vi "energy integration panel.vi"() -> ()   [LabVIEW 2017]
uses:
  control panel globals.vi
panel:
  out "fraction of energy lost/\nhalf cycle":dbl format="%_3e"
  out "adjusted energy/pulse":dbl format="%.3p"
  out "adjusted electromagnet energy":dbl format="%.3p"
  in  "coil adjustment":dbl=1.0
  out "starting energy":dbl format="%.3p"
  out "final energy":dbl format="%.3p"
  out "average energy":dbl format="%.3p"
  out "loss + change":dbl format="%.3p"
  out "energy change":dbl format="%.3p"
  out "electromagnet\nenergy":dbl format="%.3p"
  out "energy loss":dbl format="%.3p"
  out "elapsed time":dbl
  out "half cycles counted":dbl
  out "z0 from B0":dbl
  out "loss+change /hc":dbl format="%_3p"
  out "energy change/hc":dbl format="%_3p"
  out "electromagnet \nenergy/pulse":dbl format="%_3p"
  out "energy loss/hc":dbl format="%_3p"
  out "measurement":T1 {"Uavg" format="%_3p"; "Uloss" format="%_3p"; "Uloss_avg" format="%_3p"; "Upulse" format="%_3p"; "Upulse_avg" format="%_3p"; "DeltaU" format="%_3p"; "DeltaU_avg" format="%_3g"}
  in  "stop counting":bool
  in  "start counting":bool
  in  "lifetime with no drive (s)":dbl=1000.0
  in  "take snapshot":bool
  out "pulse statistics":T2 {"timing error" format="%#.3p"}
  # "totals"
  # "per 1/2 cycle"
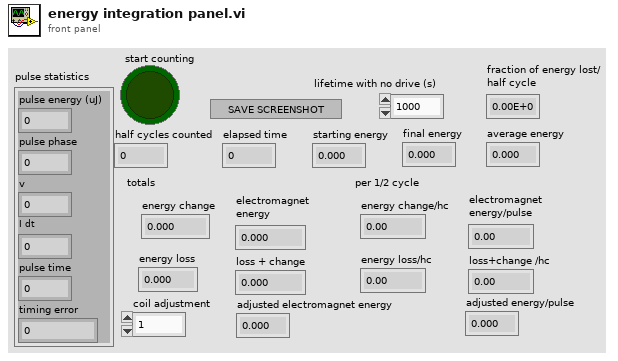
[diagram p1: front panel]
types:
  T1 = cluster{"Uavg":dbl, "Uloss":dbl, "Uloss_avg":dbl, "Upulse":dbl, "Upulse_avg":dbl, "DeltaU":dbl, "DeltaU_avg":dbl}
  T2 = cluster{"pulse energy (uJ)":sgl, "pulse phase":dbl, "v":dbl, "I dt":dbl, "pulse time":dbl, "timing error":dbl}
  T3 = cluster{"integrated pulse energy":dbl, "integrated amplitude squared":dbl, "integrated time":dbl, "integrated number of crossings":dbl, "starting amplitude squared":dbl, "final amplitude squared":dbl}
  T4 = cluster{"recent crossing":dbl, "prev crossing":dbl, "crossing-2":dbl, "number of crossings":i32, "period":dbl, "new crossing":bool, "new odd crossing":bool}
  T5 = typedef "magnetic field fit.ctl" = cluster{"a":dbl, "b":dbl, "theta":dbl, "scaling":dbl, "tilt_x":dbl, "tilt_y":dbl, "bx_offset":dbl, "by_offset":dbl, "bz_offset":dbl, "x_offset":dbl, "y_offset":dbl}
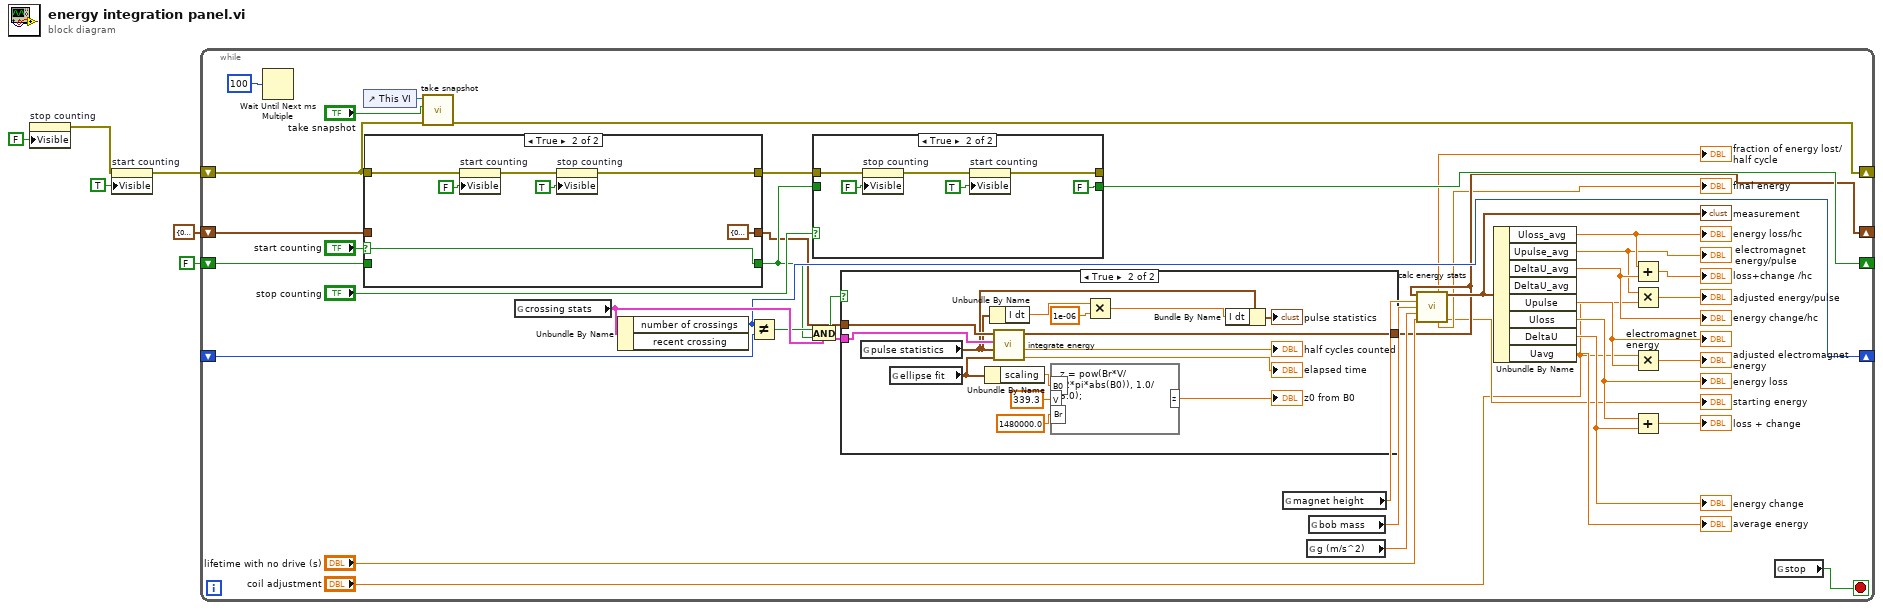
[diagram p0: block diagram]
diagram:
  n1 = property on="stop counting" class="Bool"("Visible"=FALSE) -> (error out=w4:errorcluster)  [unwired: 2 in, 1 out]
  n2 = property on="start counting" class="Bool"(error in=w4, "Visible"=TRUE) -> (error out=w3:errorcluster)  [unwired: 1 in, 1 out]
  n3 = while {
    shift-right: [w42] -> _
    shift-left: w3 -> [w36]
    shift-right: [w39] -> _
    shift-left: _ -> [w38]
    shift-right: [w15] -> _
    shift-left: T3 {"integrated pulse energy"=0.0, "integrated amplitude squared"=0.0, "integrated time"=0.0, "integrated number of crossings"=0.0, "starting amplitude squared"=0.0, "final amplitude squared"=0.0} ("integration cluster") -> [w33]
    shift-right: [w32] -> _
    shift-left: FALSE -> [w31]
    stop <- w45 stop-if-true
    n4 = Wait Until Next ms Multiple(millisecond multiple=u32 100) -> ()  [unwired: 1 out]
    n5 = control-ref of="This VI"() -> (w43:refnum<vi>)
    n6 = case shown="True" "start counting" {
      selector: "start counting" -> [_ w59]
      tunnel: [w57 T3 {"integrated pulse energy"=0.0, "integrated amplitude squared"=0.0, "integrated time"=0.0, "integrated number of crossings"=0.0, "starting amplitude squared"=0.0, "final amplitude squared"=0.0} ("integration cluster")] -> w28
      tunnel: w33 -> [w57 _]
      tunnel: w36 -> [w55 w62]
      tunnel: [w55 w60] -> w35
      tunnel: [w56 w59] -> w29
      tunnel: w31 -> [w56 _]
      frame False {
      }
      frame True {
        n7 = property on="start counting" class="Bool"(error in=w62, "Visible"=FALSE) -> (error out=w61:errorcluster)  [unwired: 1 in, 1 out]
        n8 = property on="stop counting" class="Bool"(error in=w61, "Visible"=TRUE) -> (error out=w60:errorcluster)  [unwired: 1 in, 1 out]
      }
    }
    n9 = call "take snapshot.vi"("error in (no error)"=w36, "take snapshot"="take snapshot", "vi ref"=w43) -> ("error out"=w42:errorcluster)  [unwired: 8 in]
    n10 = global read "control panel globals.vi" "crossing stats"() -> (w46:T4)
    n11 = Unbundle By Name(w46) -> ("number of crossings"=w39:i32)  [unwired: 1 out]
    n12 = Not Equal?(x=w39, y=w38) -> (x != y?=w40:bool)
    n13 = And(x=w40, y=w29) -> (x .and. y?=w30:bool)
    n14 = case shown="True" "stop counting" {
      tunnel: w35 -> [w47 w51]
      tunnel: [w47 w50] -> _
      tunnel: w29 -> [w48 _]
      tunnel: [w48 FALSE] -> w32
      frame False {
      }
      frame True {
        n15 = property on="stop counting" class="Bool"(error in=w51, "Visible"=FALSE) -> (error out=w52:errorcluster)  [unwired: 1 in, 1 out]
        n16 = property on="start counting" class="Bool"(error in=w52, "Visible"=TRUE) -> (error out=w50:errorcluster)  [unwired: 1 in, 1 out]
      }
    }
    n17 = case shown="True" w30 {
      tunnel: w46 -> [_ w80]
      tunnel: w28 -> [w65 w79]
      tunnel: [w65 w78] -> w15
      frame False {
      }
      frame True {
        n18 = global read "control panel globals.vi" "pulse statistics"() -> (w69:T2)
        n19 = global read "control panel globals.vi" "ellipse fit"() -> (w71:T5)
        n20 = Unbundle By Name(w71) -> ("scaling"=w75:dbl)
        n21 = Unbundle By Name(w69) -> ("I dt"=w68:dbl)
        n22 = call "integrate energy.vi"("ellipse fit"=w71, "pulse statistics"=w69, "crossing stats"=w80, "integration cluster"=w79) -> ("elapsed time"=→"elapsed time":dbl, "half cycles counted"=→"half cycles counted":dbl, "integration cluster out"=w78:T3)  [unwired: 5 in]
        n23 = formula code="z = pow(Br*V/(2*pi*abs(B0)), 1.0/3.0);"("B0"=w75, "V"=339.3 ("input variable"), "Br"=1480000.0 ("input variable")) -> ("z"=→"z0 from B0":dbl)
        n24 = Multiply(x=w68, y=1e-06) -> (x*y=w66:dbl)
        n25 = Bundle By Name(cluster=w69, "I dt"=w66) -> (→"pulse statistics":T2)
      }
    }
    n26 = global read "control panel globals.vi" "magnet height"() -> (w21:dbl)
    n27 = global read "control panel globals.vi" "g (m/s^2)"() -> (w20:dbl)
    n28 = global read "control panel globals.vi" "bob mass"() -> (w22:dbl)
    n29 = call "calc energy stats.vi"("integration cluster"=w15, "z0"=w21, "m"=w22, "g"=w20, "lifetime"="lifetime with no drive (s)") -> ("loss rate"=→"fraction of energy lost/\nhalf cycle":dbl, "output cluster"=w26:T1, "Ufinal"=→"final energy":dbl, "Uinit"=→"starting energy":dbl)  [unwired: 4 in, 3 out]
    "measurement" <- w26
    n30 = Unbundle By Name(w26) -> ("Uloss_avg"=w25:dbl, "Upulse_avg"=w9:dbl, "DeltaU_avg"=w24:dbl, "Upulse"=w11:dbl, "Uloss"=w19:dbl, "DeltaU"=w18:dbl, "Uavg"=→"average energy":dbl)  [unwired: 1 out]
    "energy loss/hc" <- w25
    "electromagnet \nenergy/pulse" <- w9
    "energy change/hc" <- w24
    "energy loss" <- w19
    "energy change" <- w18
    "electromagnet\nenergy" <- w11
    n31 = Add(x=w25, y=w24) -> (x+y=→"loss+change /hc":dbl)
    n32 = Multiply(x=w9, y="coil adjustment") -> (x*y=→"adjusted energy/pulse":dbl)
    n33 = Multiply(x="coil adjustment", y=w11) -> (x*y=→"adjusted electromagnet energy":dbl)
    n34 = Add(x=w19, y=w18) -> (x+y=→"loss + change":dbl)
    n35 = global read "control panel globals.vi" "stop"() -> (w45:bool)
  }
